vi "Open Viewer.vi"(8 "error in (no error)":errorcluster) -> (0 "error out":errorcluster)   [LabVIEW 2012, in "Error Logger.lvclass"]
uses:
  Error Logger.lvclass
  Error Logger.lvclass/Error Logger.ctl
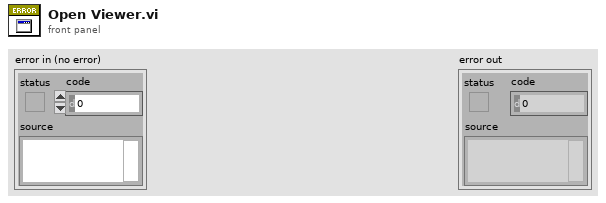
[diagram p1: front panel]
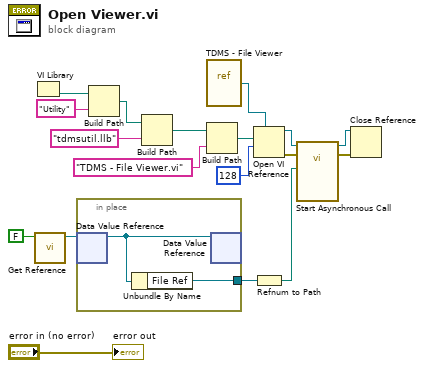
[diagram p0: block diagram]
diagram:
  n1 = VI Library() -> (path=w14:path)
  n2 = call "Get Reference.vi"("Init?"=FALSE) -> ("DVR"=w16:refnum<data-value>)  [unwired: 9 in, 1 out]
  n3 = in-place {
    in-place-border: [w19] -> w6
    n4 = in-place-dvr #1(w16) -> (w20:refnum<class "Error Logger.lvclass">)  [unwired: 1 out]
    n5 = Unbundle By Name(w20) -> ("File Ref"=w19:refnum<k34>)
    n6 = in-place-dvr #1(w20) -> ()  [unwired: 2 out]
  }
  n7 = Build Path(base path=w14, name or relative path="Utility") -> (appended path=w12:path)
  n8 = Build Path(base path=w12, name or relative path="tdmsutil.llb") -> (appended path=w10:path)
  n9 = vi-ref <vilib>:"TDMS - File Viewer.vi"() -> (w15:refnum<vi>)
  n10 = Build Path(base path=w10, name or relative path="TDMS - File Viewer.vi") -> (appended path=w8:path)
  n11 = Open VI Reference(type specifier VI Refnum (for type only)=w15, vi path=w8, options=128) -> (vi reference=w7:refnum<vi>, error out=w1:errorcluster)  [unwired: 3 in]
  n12 = Refnum to Path(1:w6) -> (0:w5:path)
  n13 = call-by-ref "Start Asynchronous Call"(reference=w7, error in=w1, "file path"=w5) -> (reference out=w3:refnum<vi>, error out=w2:errorcluster)  [unwired: 5 in, 2 out]
  n14 = Close Reference(reference=w3, error in (no error)=w2) -> ()  [unwired: 1 out]
  "error out" <- "error in (no error)"
